vi "MoistureDetection.vi"() -> ()   [LabVIEW 2023]
uses:
  Arduino DHT11/DHTXX.lvlib
  <vilib>/LabVIEW Interface for Arduino/LabVIEW Interface for Arduino.lvlib
panel:
  in  "Stop Button":bool
  in  "VISA resource":refnum<visa-resource-name>
  out "Humidity \nGraph":dbl(graph)
  out "Temperature \nGraph":dbl(graph)
  out "Humidity":dbl(slide) scale=0.0..100.0
  out "Temperature":dbl(slide) scale=0.0..50.0
  # "PLANT CARE SYSTEM"
  # "HUMIDITY PANEL"
  # "TEMPERATURE PANEL"
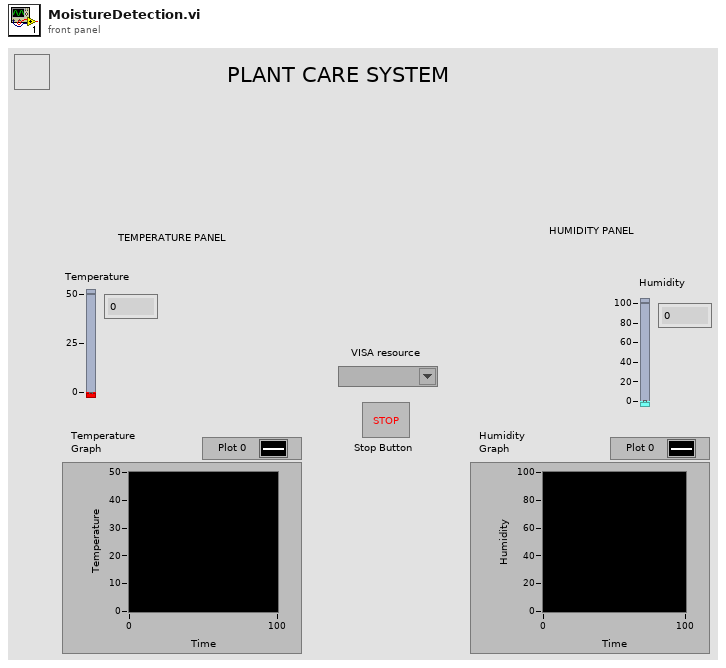
[diagram p1: front panel]
types:
  T1 = typedef "LabVIEW Interface for Arduino.lvlib/Arduino Resource.ctl" = cluster{"VISA resource":refnum<visa-resource-name>, "Board Type":T2, "Connection Type":enum8{"USB / Serial"}, "Bytes Per Packet (15)":u8}
  T2 = typedef "LabVIEW Interface for Arduino.lvlib/Board Type.ctl" = enum16{"Uno", "Dimuelanove w/Atmega 328", "Mega 2560"}
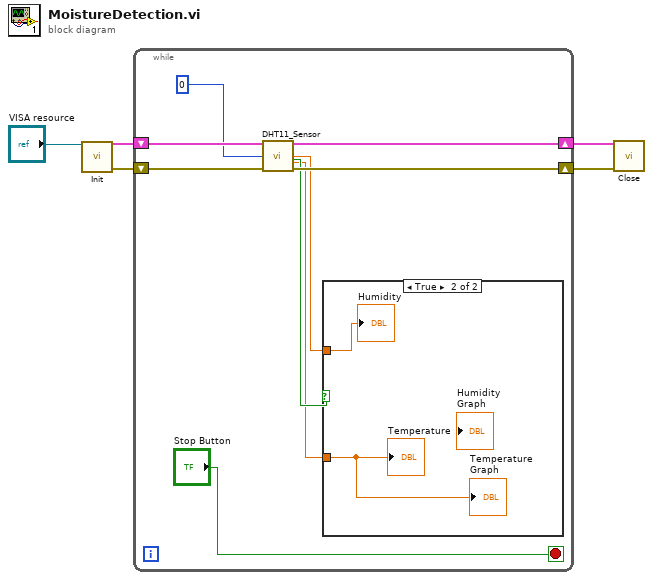
[diagram p0: block diagram]
diagram:
  n1 = call <vilib>:"Init.vi"("VISA resource"="VISA resource") -> ("Arduino Resource"=w4:T1, "error out"=w3:errorcluster)  [unwired: 17 in]
  n2 = while {
    shift-right: [w14] -> w5
    shift-left: w4 -> [w13]
    shift-right: [w11] -> w2
    shift-left: w3 -> [w12]
    stop <- "Stop Button" stop-if-true
    n3 = call "DHT11_Sensor.vi"("Arduino Resource"=w13, "Pin"=u8 0, "error in (no error)"=w12) -> ("Arduino Resource"=w14:T1, "Successful?"=w9:bool, "Relative Humidity"=w8:dbl, "Temperature (°C)"=w7:dbl, "error out"=w11:errorcluster)  [unwired: 8 in]
    n4 = case shown="True" w9 {
      tunnel: w8 -> [_ w16]
      tunnel: w7 -> [_ w15]
      frame False {
      }
      frame True {
        "Humidity" <- w16
        "Temperature" <- w15
        "Temperature \nGraph" <- w15
      }
    }
  }
  n5 = call <vilib>:"Close.vi"("Arduino Resource"=w5, "error in"=w2) -> ()  [unwired: 13 in, 1 out]
